vi "subVI_velocitymode_rev2.vi"(7 "CH":bool[](array[boolean])=[FALSE, FALSE, TRUE, FALSE, FALSE, TRUE, FALSE, FALSE, FALSE, FALSE, FALSE, FALSE, FALSE, FALSE, FALSE, FALSE], 9 "DAC1":bool[](array[boolean]), 10 "error in":errorcluster, 11 "FPGA VI Reference In":refnum<k20>) -> (0 "FPGA VI Reference Out":refnum<k20>, 1 "i":u32, 2 "GAIN":i16, 3 "UNI":i16, 4 "error out":errorcluster)   [LabVIEW 2018]
uses:
  <vilib>/Utility/error.llb/Error Cluster From Error Code.vi
  <vilib>/rvi/errors/niLvFpgaAdjustHostInterfaceError.vi
  <vilib>/rvi/interface/nirviReadWriteControl/nirviReadWriteControl.xnode
  NiFpgaLv.dll
  <vilib>/rvi/interface/Simulation/niFpgaSimulationCallBeginRW.vi
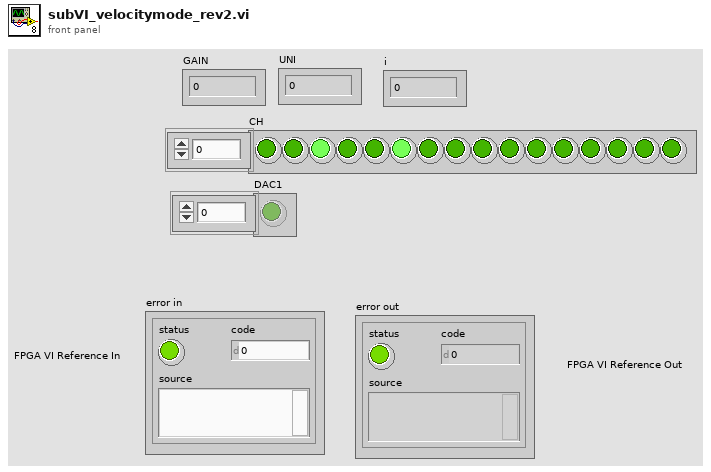
[diagram p1: front panel]
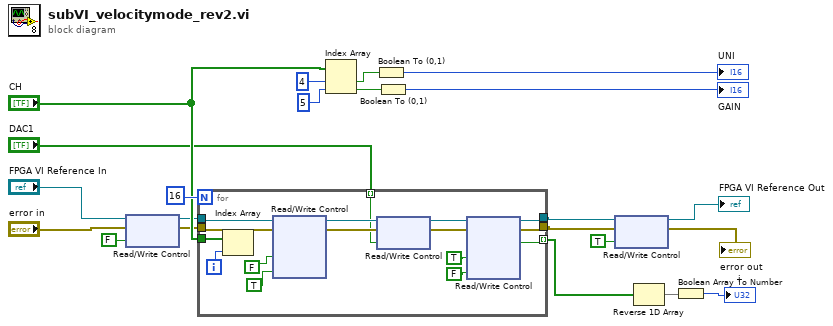
[diagram p0: block diagram]
diagram:
  n1 = xnode "Read/Write Control"("FPGA VI Reference In"="FPGA VI Reference In", "error in"="error in", "CS"=FALSE) -> ("FPGA VI Reference Out"=w2:refnum<k20>, "error out"=w1:errorcluster)
  n2 = for {
    N: 16 -> [_]
    tunnel: w2 -> [w30]
    tunnel: w1 -> [w29]
    tunnel: [w27] -> w16 mode=indexing
    tunnel: [w26] -> w20
    tunnel: [w25] -> w19
    tunnel: "CH" -> [w24]
    tunnel: "DAC1" -> [w23] mode=indexing
    i -> [w28]
    n3 = Index Array(array=w24, index=w28) -> ()  [unwired: 1 out]
    n4 = xnode "Read/Write Control"("FPGA VI Reference In"=w30, "error in"=w29, "CLK2"=FALSE ("CLK"), "CLK1"=TRUE ("CLK")) -> ("FPGA VI Reference Out"=w36:refnum<k20>, "error out"=w35:errorcluster)  [unwired: 1 in]
    n5 = xnode "Read/Write Control"("FPGA VI Reference In"=w36, "error in"=w35, "MOSI2"=w23) -> ("FPGA VI Reference Out"=w34:refnum<k20>, "error out"=w33:errorcluster)
    n6 = xnode "Read/Write Control"("FPGA VI Reference In"=w34, "error in"=w33, "CLK2"=TRUE, "CLK1"=FALSE) -> ("FPGA VI Reference Out"=w26:refnum<k20>, "error out"=w25:errorcluster, "MISO1"=w27:bool)
  }
  n7 = Index Array(array="CH", index #1=4 ("index"), index #2=5 ("index")) -> (element #1=w14:bool, element #2=w13:bool)
  n8 = Boolean To (0,1)(Boolean=w14) -> (0, 1=→"UNI":i16)
  n9 = Boolean To (0,1)(Boolean=w13) -> (0, 1=→"GAIN":i16)
  n10 = xnode "Read/Write Control"("FPGA VI Reference In"=w20, "error in"=w19, "CS"=TRUE) -> ("FPGA VI Reference Out"=→"FPGA VI Reference Out":refnum<k20>, "error out"=→"error out":errorcluster)
  n11 = Reverse 1D Array(array=w16) -> (reversed array=w15:bool[])
  n12 = Boolean Array To Number(Boolean array=w15) -> (number=→"i":u32)
